vi "MovePoint.vi"(4 "FlipY":bool, 6 "FlipX":bool, 7 "Controls Reference Out":T3, 8 "error in (no error)":errorcluster, 9 "Index":i32, 10 "Settings In":T6={"Calibration Input"=[], "CalibrationResults"={"Center in Pixels"=[374.0120339529387, 375.46592887074246], "Angle"=0.022945275255000355, "Pixels/MHz X"=0.0, "Pixels/MHz Y"=0.0}, "Highlight"=[], "Running Script"=refnum}, 11 "Queues Out":T1) -> (0 "error out":errorcluster)   [LabVIEW 2017]
uses:
  ExperimentVariables.ctl
  AODControl/AODControlFiles/InterfaceReferences.ctl
  AODControl/AODControlFiles/LoadControl.ctl
  AODControl/AODControlFiles/ExitButton.ctl
  ImageAcquisitionProgram/ImageAcquisitionLibrary/References.ctl
  SubVIQueues.ctl
  AODControl/MessageQueue/QueueOperations/All Message Queues.ctl
  AODControl/MessageQueue/QueueOperations/Message Cluster.ctl
  AODControl/AODControlFiles/AODPointDefinition.ctl
  MessageQueue/QueueOperations/Enqueue Message (Single).vi
  MessageQueue/MessageQueue.lvlib
  AODControl/AODControl.lvlib
  AODControl/MessageQueue/MessageQueue.lvlib
  ImageAcquisitionProgram/ImageAcquisitionLibrary/ImageAcquisitionLibrary.lvlib
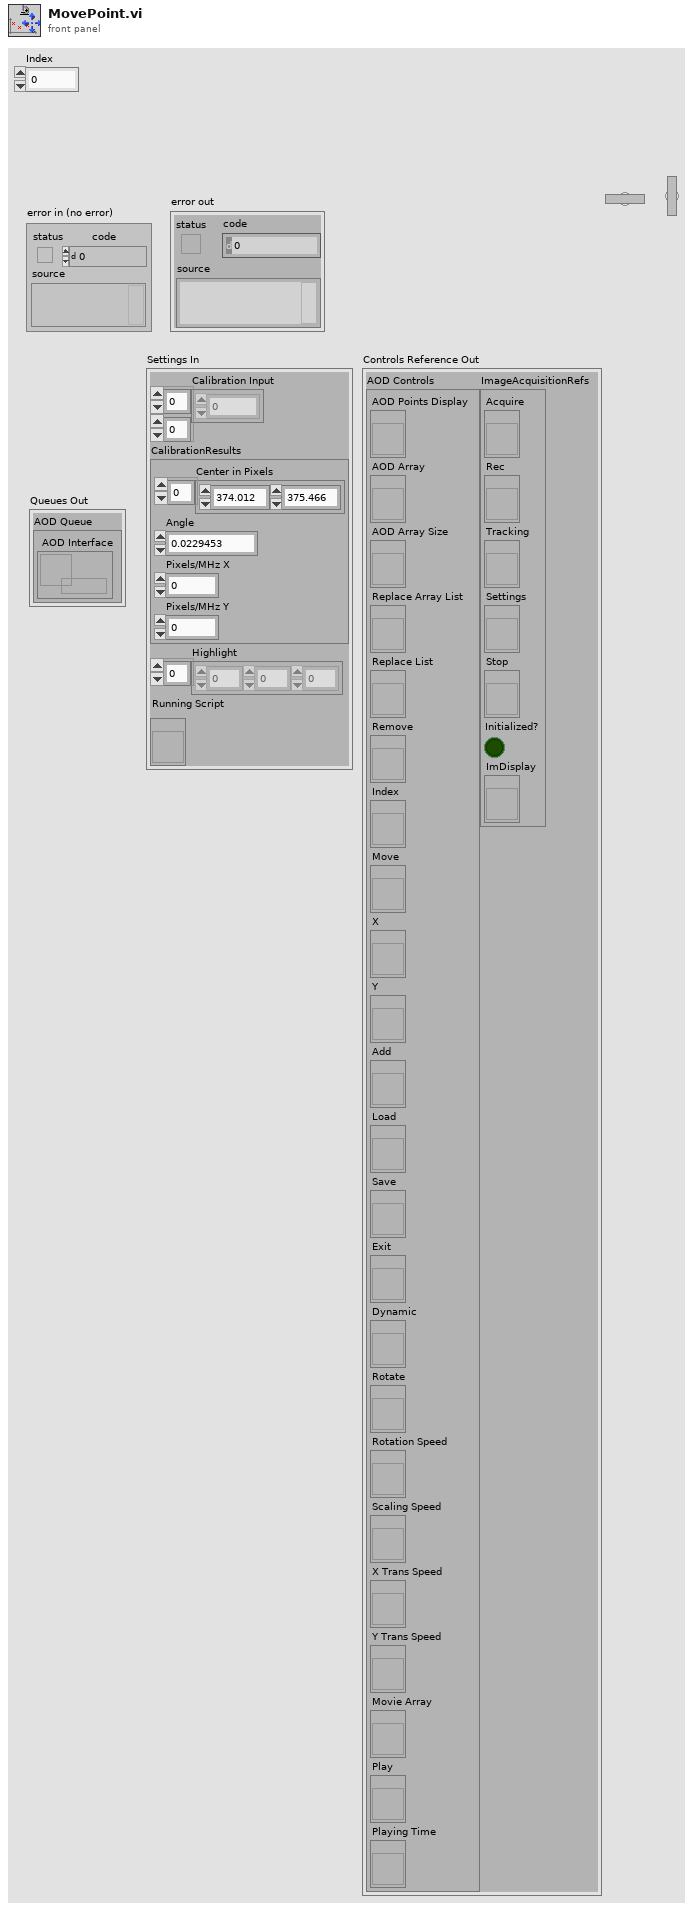
[diagram p1: front panel]
types:
  T1 = typedef "SubVIQueues.ctl" = cluster{"AOD Queue":T2}
  T2 = typedef "AODControl.lvlib/MessageQueue.lvlib/All Message Queues.ctl" = cluster{" AOD Interface":refnum<queue>}
  T3 = typedef "ExperimentControls" = cluster{"AOD Controls":T4, "ImageAcquisitionRefs":T5}
  T4 = typedef "AODControl.lvlib/InterfaceReferences.ctl" = cluster{"AOD Points Display":refnum<vi>, "AOD Array":refnum<vi>, "AOD Array Size":refnum<vi>, "Replace Array List":refnum<vi>, "Replace List":refnum<vi>, "Remove":refnum<vi>, "Index":refnum<vi>, "Move":refnum<vi>, "X":refnum<vi>, "Y":refnum<vi>, "Add":refnum<vi>, "Load":refnum<vi>, "Save":refnum<vi>, "Exit":refnum<vi>, "Dynamic":refnum<vi>, "Rotate":refnum<vi>, "Rotation Speed":refnum<vi>, "Scaling Speed":refnum<vi>, "X Trans Speed":refnum<vi>, "Y Trans Speed":refnum<vi>, "Movie Array":refnum<vi>, "Play":refnum<vi>, "Playing Time":refnum<vi>}
  T5 = typedef "ImageAcquisitionLibrary.lvlib/References.ctl" = cluster{"Acquire":refnum<vi>, "Rec":refnum<vi>, "Tracking":refnum<vi>, "Settings":refnum<vi>, "Stop":refnum<vi>, "Initialized?":bool, "ImDisplay":refnum<vi>}
  T6 = typedef "ExperimentVariables.ctl" = cluster{"Calibration Input":i32[][], "CalibrationResults":cluster{"Center in Pixels":dbl[], "Angle":dbl, "Pixels/MHz X":dbl, "Pixels/MHz Y":dbl}, "Highlight":i32[], "Running Script":refnum<vi>}
  T7 = typedef "AODControl.lvlib/AODPointDefinition.ctl" = cluster{"Freq X":dbl, "Freq Y":dbl, "Index":i32, "Ampitude":dbl}
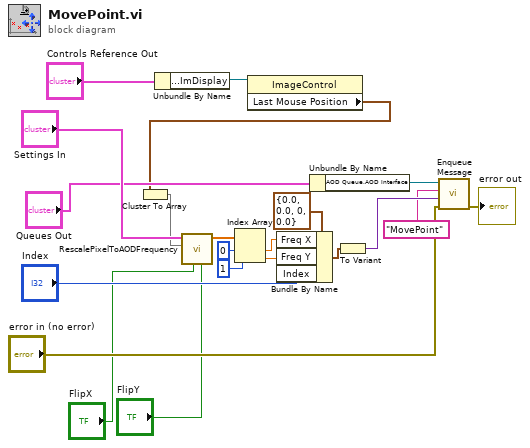
[diagram p0: block diagram]
diagram:
  n1 = Unbundle By Name("Controls Reference Out") -> ("ImageAcquisitionRefs.ImDisplay"=w5:refnum<vi>)
  n2 = property class="ImageControl"(reference=w5) -> ("Last Mouse Position"=w4:cluster{"X":i32, "Y":i32})  [unwired: 1 in, 2 out]
  n3 = Cluster To Array(cluster=w4) -> (array=w20:i32[])
  n4 = call "RescalePixelToAODFrequency.vi"("FlipY"="FlipY", "FlipX"="FlipX", "Pixels"=w20, 11:"Settings In") -> ("Array"=w16:dbl[])  [unwired: 7 in]
  n5 = Index Array(array=w16, index #1=0 ("index"), index #2=1 ("index")) -> (element #1=w14:dbl, element #2=w15:dbl)
  n6 = Bundle By Name(cluster=T7 {"Freq X"=0.0, "Freq Y"=0.0, "Index"=0, "Ampitude"=0.0} ("Cluster"), "Freq X"=w14, "Freq Y"=w15, "Index"="Index") -> (w18:T7)
  n7 = Unbundle By Name("Queues Out") -> ("AOD Queue.AOD Interface"=w10:refnum<queue>)
  n8 = To Variant(anything=w18) -> (Variant=w19:variant)
  n9 = call-poly "Enqueue Message.vi"("error in (no error)"="error in (no error)", "Message Data"=w19, "Message"="MovePoint", "Message Queue"=w10) -> ("error out"=→"error out":errorcluster)  [unwired: 6 in, 1 out]
